vi "Dialog - Prompt Open Style.vi"(8 "error in (no error)":errorcluster, 10 "Include active book option?":bool) -> (0 "error out":errorcluster, 3 "Open Style":T1(ring))   [LabVIEW 2016, in "Excel.lvclass"]
uses:
  Excel.lvclass
panel:
  in  "Tab Control":enum32{"No Active Book", "Active Book"}(tab)
  in  "Btn_Existing 2":bool
  in  "Btn_New 2":bool
  in  "Btn_Existing":bool
  in  "Btn_New":bool
  in  "Btn_Active":bool
  # "Attempting to access an Excel Workbook.\nChoose whether to open an..."
  # "Attempting to access an Excel Workbook.\nChoose whether to open an..."
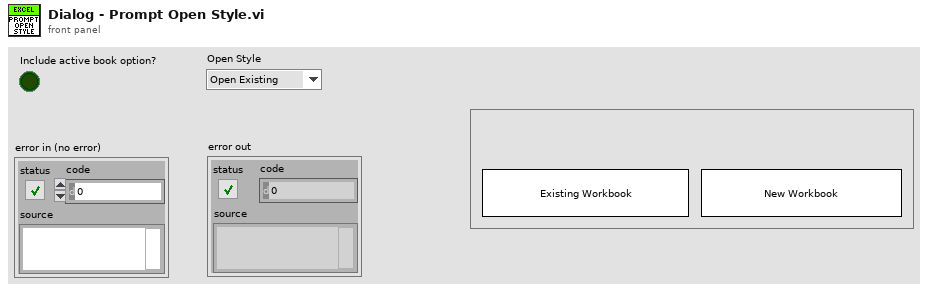
[diagram p1: front panel]
types:
  T1 = enum16{"Open Existing", "Open Active", "Open New", "Cancelled"}
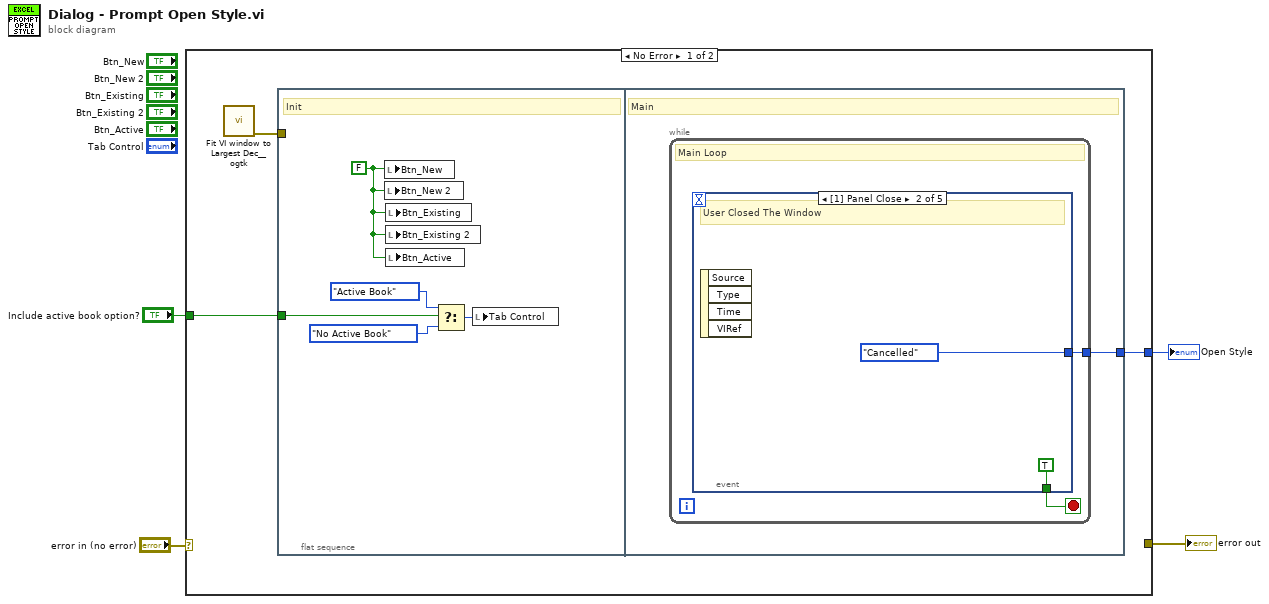
[diagram p0: block diagram]
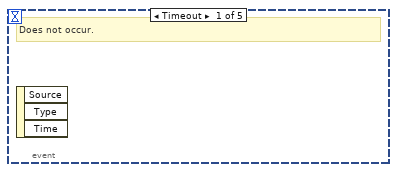
[diagram p2: hidden frame]
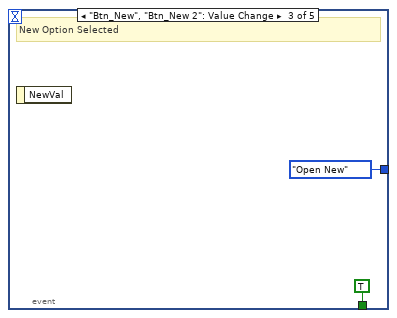
[diagram p3: hidden frame]
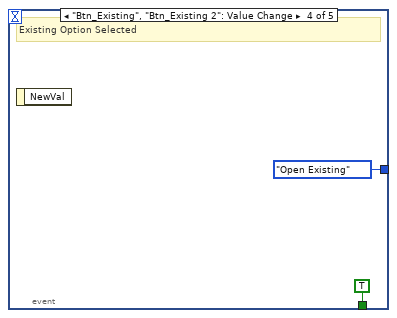
[diagram p4: hidden frame]
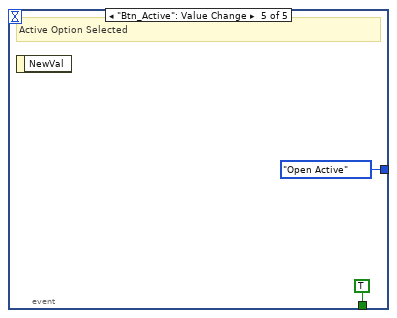
[diagram p5: hidden frame]
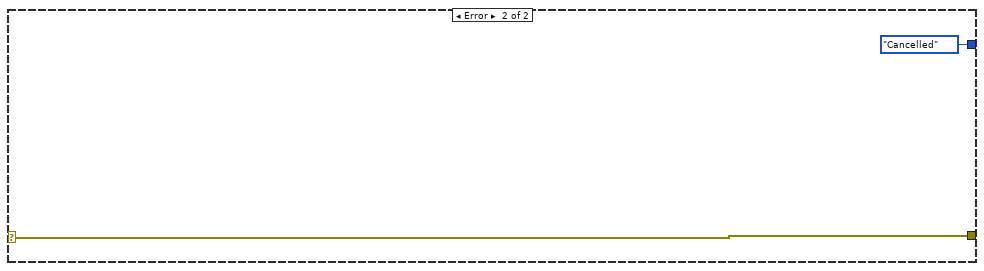
[diagram p6: hidden frame]
diagram:
  n1 = case shown="No Error" "error in (no error)" {
    selector: "error in (no error)" -> [_ w25]
    tunnel: [_ w25] -> w3
    tunnel: "Include active book option?" -> [w7 _]
    tunnel: [w6 T1."Cancelled" ("Open Style")] -> w1
    frame No Error {
      n2 = call <userlib>:"Fit VI window to Largest Dec__ogtk.vi"() -> ("error out"=w5:errorcluster)  [unwired: 6 in, 1 out]
      n3 = flat-sequence {
        tunnel: w7 -> [w12]
        tunnel: w5 -> [_]
        tunnel: [w13] -> w6
        frame #0 {
          w8 = FALSE ("Btn_New")
          # "Init"
          n4 = local write "Btn_New"(w8) -> ()
          n5 = local write "Btn_New 2"(w8) -> ()
          n6 = local write "Btn_Existing"(w8) -> ()
          n7 = local write "Btn_Existing 2"(w8) -> ()
          n8 = local write "Btn_Active"(w8) -> ()
          n9 = Select(t=enum32{"No Active Book", "Active Book"}."Active Book" ("Tab Control"), s=w12, f=enum32{"No Active Book", "Active Book"}."No Active Book" ("Tab Control")) -> (s? t:f=w9:enum32{"No Active Book", "Active Book"})
          n10 = local write "Tab Control"(w9) -> ()
        }
        frame #1 {
          # "Main"
          n11 = while {
            tunnel: [w14] -> w13
            stop <- w15 stop-if-true
            # "Main Loop"
            n12 = event shown="[1] Panel Close" {
              selector: _ -> [_ _ _ _ _]
              dyn-events: _ -> [_ _ _ _ _]
              timeout: _ -> [_ _ _ _ _]
              tunnel: [_ TRUE TRUE TRUE TRUE] -> w15
              tunnel: [_ T1."Cancelled" ("Open Style") T1."Open New" ("Open Style") T1."Open Existing" ("Open Style") T1."Open Active" ("Open Style")] -> w14
              event Timeout {
                # "Does not occur."
                n13 = event-data() -> ()  [unwired: 1 in, 3 out]
              }
              event Panel Close {
                # "User Closed The Window"
                n14 = event-data() -> ()  [unwired: 1 in, 4 out]
              }
              event "Btn_New", "Btn_New 2": Value Change {
                # "New Option Selected"
                n15 = event-data() -> ()  [unwired: 1 in, 1 out]
              }
              event "Btn_Existing", "Btn_Existing 2": Value Change {
                # "Existing Option Selected"
                n16 = event-data() -> ()  [unwired: 1 in, 1 out]
              }
              event "Btn_Active": Value Change {
                # "Active Option Selected"
                n17 = event-data() -> ()  [unwired: 1 in, 1 out]
              }
            }
          }
        }
      }
    }
    frame Error {
    }
  }
  "error out" <- w3
  "Open Style" <- w1
